vi "SET DO AO PLC 1.vi"(10 "USCITE PLC":T1, 11 "Q":string="PLC_1_Q") -> ()   [LabVIEW 2019]
uses:
  Uscite PLC 1.ctl
  controls/statoAO_plc_1.ctl
  StatoDO_PLC_1.ctl
  TypeDef_PLC_Q.ctl
panel:
  # "StatoDO_PLC.ctlUSCITE PLC : TYPE DEF"
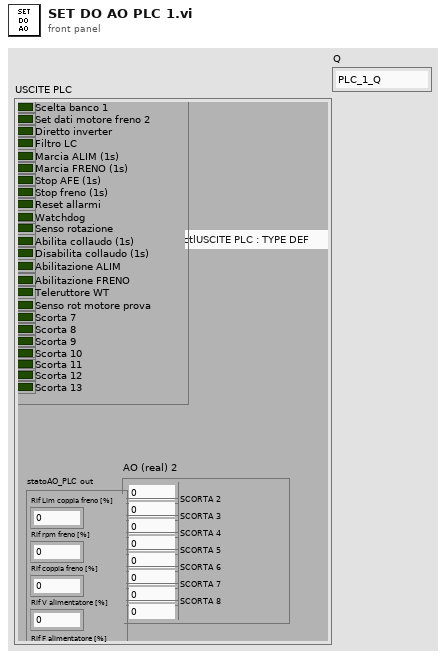
[diagram p1: front panel]
types:
  T1 = typedef "Uscite PLC 1.ctl" = cluster{"AO (real) 2":cluster{"SCORTA 1":dbl, "SCORTA 2":dbl, "SCORTA 3":dbl, "SCORTA 4":dbl, "SCORTA 5":dbl, "SCORTA 6":dbl, "SCORTA 7":dbl, "SCORTA 8":dbl}, "statoAO_PLC out":T2, "DO (bit)":T3}
  T2 = typedef "statoAO_plc_1.ctl" = cluster{"Rif Lim coppia freno [%]":dbl, "Rif rpm freno [%]":dbl, "Rif coppia freno [%]":dbl, "Rif V alimentatore [%]":dbl, "Rif F alimentatore [%]":dbl}
  T3 = typedef "StatoDO_PLC_1.ctl" = cluster{"Scelta banco 1":bool, "Set dati motore freno 2":bool, "Diretto inverter":bool, "Filtro LC":bool, "Marcia ALIM (1s)":bool, "Marcia FRENO (1s)":bool, "Stop AFE (1s)":bool, "Stop freno (1s)":bool, "Reset allarmi":bool, "Watchdog":bool, "Senso rotazione":bool, "Abilita collaudo (1s)":bool, "Disabilita collaudo (1s)":bool, "Abilitazione ALIM":bool, "Abilitazione FRENO":bool, "Teleruttore WT":bool, "Senso rot motore prova":bool, "Scorta 7":bool, "Scorta 8":bool, "Scorta 9":bool, "Scorta 10":bool, "Scorta 11":bool, "Scorta 12":bool, "Scorta 13":bool}
  T4 = typedef "TypeDef_PLC_Q.ctl" = cluster{"Message":string, "Data":variant}
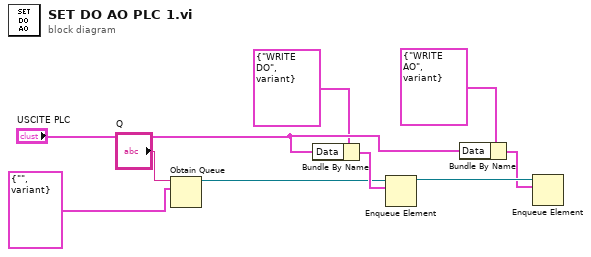
[diagram p0: block diagram]
diagram:
  n1 = Obtain Queue(name (unnamed)="Q", element data type=T4 {"Message"="", "Data"=variant}) -> (queue out=w2:refnum<queue>)  [unwired: 3 in, 2 out]
  n2 = Bundle By Name(cluster=T4 {"Message"="WRITE DO", "Data"=variant}, "Data"="USCITE PLC") -> (w4:T4)
  n3 = Enqueue Element(queue=w2, element=w4) -> (queue out=w8:refnum<queue>)  [unwired: 2 in, 2 out]
  n4 = Bundle By Name(cluster=T4 {"Message"="WRITE AO", "Data"=variant}, "Data"="USCITE PLC") -> (w7:T4)
  n5 = Enqueue Element(queue=w8, element=w7) -> ()  [unwired: 2 in, 3 out]
